vi "Set Default Value.vi"(9 "Default C++ Value":string, 10 "Control Ref":refnum<vi>, 11 "C String Writer in":refnum<class "C String Writer.lvclass">) -> (1 "LabVIEW Default String":string, 2 "Control Ref Dup":refnum<vi>, 3 "C String Writer out":refnum<class "C String Writer.lvclass">)   [LabVIEW 2014, in "C String Writer.lvclass"]
doc: "Copyright (c) 2016 Sze Howe Koh\n\nThis Source Code Form is subject to the terms of the Mozilla Public License, v. 2.0. If a copy of the MPL was not distributed with this file, You can obtain one at http://mozilla.org/MPL/2.0/."
uses:
  C String Writer.lvclass
  String Writer/String Writer.lvclass
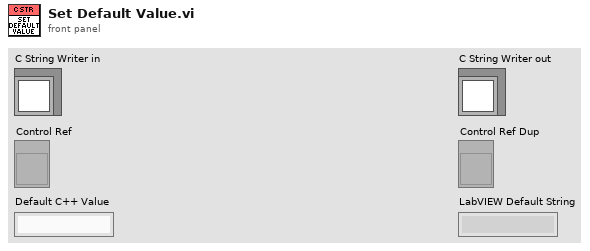
[diagram p1: front panel]
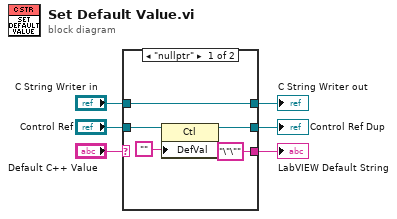
[diagram p0: block diagram]
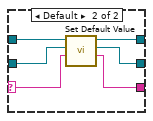
[diagram p2: hidden frame]
diagram:
  n1 = case shown="\"nullptr\"" "Default C++ Value" {
    selector: "Default C++ Value" -> [_ w12]
    tunnel: ["\"\"" ("LabVIEW Default String") w17] -> w6
    tunnel: [w9 w16] -> w5
    tunnel: [w11 w15] -> w4
    tunnel: "Control Ref" -> [w10 w14]
    tunnel: "C String Writer in" -> [w11 w13]
    frame "nullptr" {
      n2 = property class="Ctl"(reference=w10, "DefVal"="") -> (reference out=w9:refnum<vi>)  [unwired: 1 in, 1 out]
    }
    frame Default {
      n3 = call-parent "Set Default Value.vi"("Default C++ Value"=w12, "Control Ref"=w14, "String Writer in"=w13) -> ("LabVIEW Default String"=w17:string, "Control Ref Dup"=w16:refnum<vi>, "String Writer out"=w15:refnum<class "C String Writer.lvclass">)  [unwired: 6 in]
    }
  }
  "C String Writer out" <- w4
  "Control Ref Dup" <- w5
  "LabVIEW Default String" <- w6
